vi "Query DMRS For Mapping Type A.vi"(7 "BWP (BWP0)":i32(ring) items=["BWP0"], 8 "error in (no error)":errorcluster, 9 "CC (1)":T1=1, 10 "Instance (1)":T2=1, 11 "VISA resource name":refnum<visa-resource-name>) -> (0 "error out":errorcluster, 1 "Additional Position":i32, 2 "Config Type":i32, 3 "VISA resource name out":refnum<visa-resource-name>, 4 "Max Length":i32)   [LabVIEW 2020, in "Rohde&Schwarz CMWXP NR FR1 Measurement.lvlib"]
doc: "Queries the DM-RS for mapping type A. The settings apply to the <BWP> on carrier <no>.\n\nAttribute:\n-\n\nRemote-control command:\nCONFigure:NRSub:MEAS<i>[:CC<no>]:BWPart:PUSCh:DMTA?"
uses:
  <instrlib>/Rohde&Schwarz CMWXP NR FR1 Measurement/Rohde&Schwarz CMWXP NR FR1 Measurement.lvlib
  <instrlib>/Rohde&Schwarz CMWXP NR FR1 Measurement/Private/_Instance.ctl
  <instrlib>/Rohde&Schwarz CMWXP NR FR1 Measurement/Private/_Carrier Component.ctl
  <instrlib>/Rohde&Schwarz CMWXP NR FR1 Measurement/Private/rsidr_core.llb/rsidr_core.lvlib
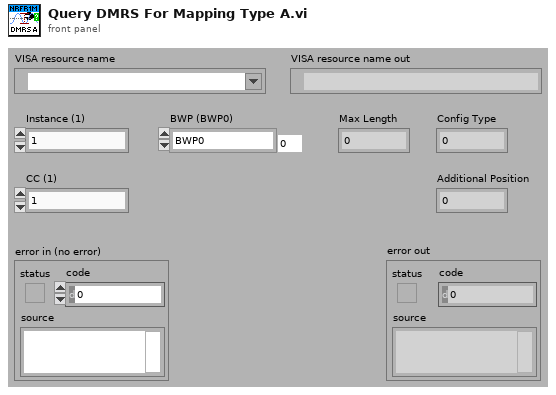
[diagram p1: front panel]
types:
  T1 = typedef "Rohde&Schwarz CMWXP NR FR1 Measurement.lvlib/_Carrier Component.ctl" = i32
  T2 = typedef "Rohde&Schwarz CMWXP NR FR1 Measurement.lvlib/_Instance.ctl" = i32
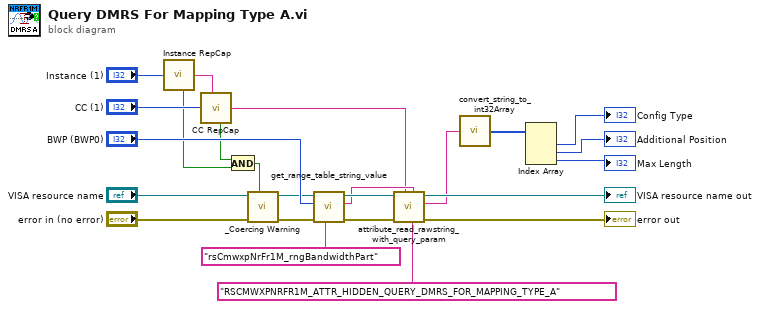
[diagram p0: block diagram]
diagram:
  n1 = call <instrlib>:"Instance RepCap.vi"("Instance In"="Instance (1)") -> ("In Range?"=w2:bool, "RepCap Identifier Out"=w24:string)  [unwired: 1 in]
  n2 = call <instrlib>:"CC RepCap.vi"("CC In"="CC (1)", "RepCap String In (\"\")"=w24) -> ("In Range?"=w1:bool, "RepCap Identifier Out"=w19:string)
  n3 = And(x=w1, y=w2) -> (x .and. y?=w3:bool)
  n4 = call <instrlib>:"_Coercing Warning.vi"("In Range?"=w3, "error in (no error)"="error in (no error)", "VISA resource name"="VISA resource name") -> ("error out"=w5:errorcluster, "VISA resource name out"=w4:refnum<visa-resource-name>)  [unwired: 7 in]
  n5 = call <instrlib>:"get_range_table_string_value.vi"("Range Table ID in"="rsCmwxpNrFr1M_rngBandwidthPart", "error in"=w5, "I32 input"="BWP (BWP0)", "VISA resource name"=w4) -> ("error out"=w22:errorcluster, "String Value out"=w20:string, "VISA resource name out"=w21:refnum<visa-resource-name>)  [unwired: 5 in]
  n6 = call <instrlib>:"attribute_read_rawstring_with_query_param.vi"("Query Parameter (None)"=w20, "Repeated Capability"=w19, "error in"=w22, "Attribute ID"="RSCMWXPNRFR1M_ATTR_HIDDEN_QUERY_DMRS_FOR_MAPPING_TYPE_A", "VISA resource name"=w21) -> ("error out"=→"error out":errorcluster, "Raw String out"=w12:string, "VISA resource name out"=→"VISA resource name out":refnum<visa-resource-name>)  [unwired: 4 in]
  n7 = call <instrlib>:"convert_string_to_int32Array.vi"("string in"=w12) -> ("int32 array out"=w11:i32[])  [unwired: 3 in, 1 out]
  n8 = Index Array(array=w11) -> (element #1=→"Config Type":i32, element #2=→"Additional Position":i32, element #3=→"Max Length":i32)  [unwired: 3 in]
